vi "Lookup Southeast.vi"() -> (3 "City":T1)   [LabVIEW 2017]
uses:
  Cities Enum.ctl
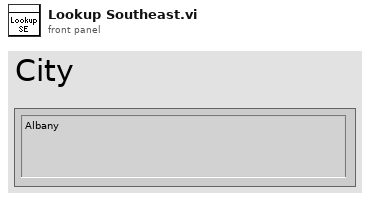
[diagram p1: front panel]
types:
  T1 = typedef "Cities Enum.ctl" = enum16{"Albany", "Baltimore", "Boston", "Buffalo", "New York", "Philadelphia", "Pittsburgh", "ME, Portland", "Washington", "Atlanta", "Charleston", "Charlotte", "Chattanooga", "Jacksonville", "Knoxville", "Miami", "Mobile", "Norfolk", "Richmond", "Tampa", "Chicago", "Cincinnati", "Cleveland", "Columbus", "Detroit", "Indianapolis", "Milwaukee", "StLouis", "Birmingham", "Dallas", "Fort Worth", "Houston", "Little Rock", "Louisville", "Memphis", "Nashville", "New Orleans", "San Antonio", "Shreveport", "Denver", "Des Moines", "Fargo", "Kansas City", "Minneapolis", "Oklahoma City", "Omaha", "Pueblo", "StPaul", "Billings", "Butte", "Casper", "Pocatello", "OR, Portland", "Rapid City", "Salt Lake City", "Seattle", "Spokane", "El Paso", "Las Vegas", "Los Angeles", "Oakland", "Phoenix", "Reno", "Sacramento", "San Diego", "San Francisco", "Tucumcari"}
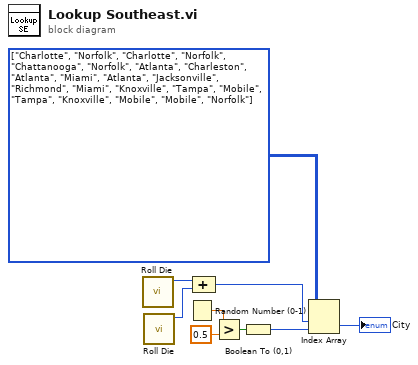
[diagram p0: block diagram]
diagram:
  w4 = T1[][] [[enum."Charlotte", enum."Norfolk"], [enum."Charlotte", enum."Norfolk"], [enum."Chattanooga", enum."Norfolk"], [enum."Atlanta", enum."Charleston"], [enum."Atlanta", enum."Miami"], [enum."Atlanta", enum."Jacksonville"], [enum."Richmond", enum."Miami"], [enum."Knoxville", enum."Tampa"], [enum."Mobile", enum."Tampa"], [enum."Knoxville", enum."Mobile"], [enum."Mobile", enum."Norfolk"]] items=["Albany", "Baltimore", "Boston", "Buffalo", "New York", "Philadelphia", "Pittsburgh", "ME, Portland", "Washington", "Atlanta", "Charleston", "Charlotte", "Chattanooga", "Jacksonville", "Knoxville", "Miami", "Mobile", "Norfolk", "Richmond", "Tampa", "Chicago", "Cincinnati", "Cleveland", "Columbus", "Detroit", "Indianapolis", "Milwaukee", "StLouis", "Birmingham", "Dallas", "Fort Worth", "Houston", "Little Rock", "Louisville", "Memphis", "Nashville", "New Orleans", "San Antonio", "Shreveport", "Denver", "Des Moines", "Fargo", "Kansas City", "Minneapolis", "Oklahoma City", "Omaha", "Pueblo", "StPaul", "Billings", "Butte", "Casper", "Pocatello", "OR, Portland", "Rapid City", "Salt Lake City", "Seattle", "Spokane", "El Paso", "Las Vegas", "Los Angeles", "Oakland", "Phoenix", "Reno", "Sacramento", "San Diego", "San Francisco", "Tucumcari"]
  n1 = call "Roll Die.vi"() -> ("Number"=w5:i32)  [unwired: 11 in]
  n2 = call "Roll Die.vi"() -> ("Number"=w6:i32)  [unwired: 11 in]
  n3 = Random Number (0-1)() -> (number: 0 to 1=w7:dbl)
  n4 = Compound Arithmetic op=ADD(w5, w6) -> (w3:i32)
  n5 = Greater?(x=w7, y=0.5) -> (0:w9:bool)
  n6 = Boolean To (0,1)(Boolean=w9) -> (0, 1=w2:i16)
  n7 = Index Array(array=w4, index (row)=w3, index (col)=w2) -> (element=→"City":T1)
